vi "Close References.vi"(8 "error in (no error)":errorcluster, 10 "VI Refnum":refnum<vi>, 11 "Variant":variant) -> (0 "error out":errorcluster)   [LabVIEW 2016, in "M1M3SupportEUI_Views.lvlib"]
uses:
  M1M3SupportEUI_Views.lvlib
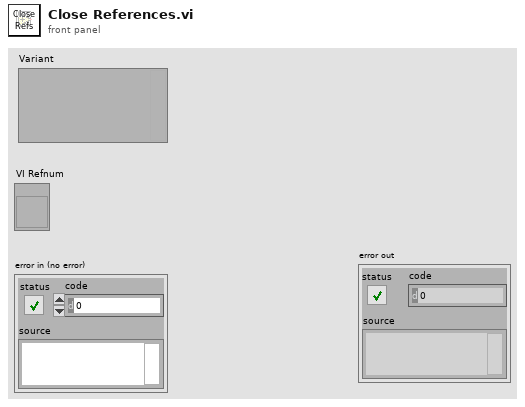
[diagram p1: front panel]
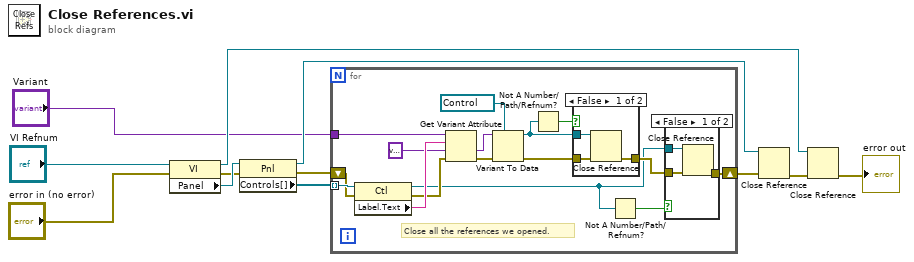
[diagram p0: block diagram]
diagram:
  n1 = property class="VI"(reference="VI Refnum", error in="error in (no error)") -> (reference out=w10:refnum<vi>, error out=w5:errorcluster, "Panel"=w6:refnum<vi>)
  n2 = property class="Pnl"(reference=w6, error in=w5) -> (reference out=w12:refnum<vi>, error out=w9:errorcluster, "Controls[]"=w11:refnum<vi>[])
  n3 = for {
    tunnel: w11 -> [w27] mode=indexing
    tunnel: "Variant" -> [w28]
    shift-right: [w17] -> w7
    shift-left: w9 -> [w25]
    # "Close all the references we opened."
    n4 = property class="Ctl"(reference=w27, error in=w25) -> (reference out=w14:refnum<vi>, error out=w24:errorcluster, "Label.Text"=w26:string)
    n5 = Get Variant Attribute(Variant=w28, name=w26, default value (empty Variant)=variant ("default value (empty variant)"), error in=w24) -> (value=w22:variant, error out=w23:errorcluster)  [unwired: 2 out]
    n6 = Variant To Data(error in=w23, type=refnum<vi> refnum ("reference out"), Variant=w22) -> (data=w16:refnum<vi>, error out=w19:errorcluster)
    n7 = Not A Number/Path/Refnum?(number/path/refnum=w16) -> (NaN/Path/Refnum?=w15:bool)
    n8 = case shown="False" w15 {
      tunnel: w19 -> [w35 w36]
      tunnel: [w34 w36] -> w18
      tunnel: w16 -> [w33 _]
      frame False {
        n9 = Close Reference(reference=w33, error in (no error)=w35) -> (error out=w34:errorcluster)
      }
      frame True {
      }
    }
    n10 = Not A Number/Path/Refnum?(number/path/refnum=w14) -> (NaN/Path/Refnum?=w13:bool)
    n11 = case shown="False" w13 {
      tunnel: w18 -> [w31 w32]
      tunnel: [w30 w32] -> w17
      tunnel: w14 -> [w29 _]
      frame False {
        n12 = Close Reference(reference=w29, error in (no error)=w31) -> (error out=w30:errorcluster)
      }
      frame True {
      }
    }
  }
  n13 = Close Reference(reference=w12, error in (no error)=w7) -> (error out=w8:errorcluster)
  n14 = Close Reference(reference=w10, error in (no error)=w8) -> (error out=→"error out":errorcluster)
